vi "Camera ROI.vi"(10 "View (%)":sgl=100.0 min=0 max=100, 11 "Crop Point":i32=60 min=0 max=160 step=1) -> (3 "Camera ROI":i32[](array[numeric]))   [LabVIEW 2012]
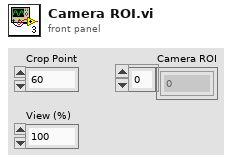
[diagram p1: front panel]
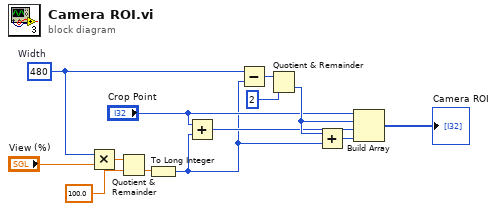
[diagram p0: block diagram]
diagram:
  w5 = 480  # Width
  n1 = Multiply(x=w5, y="View (%)") -> (x*y=w4:sgl)
  n2 = Quotient & Remainder(x=w4, y=sgl 100.0) -> (floor(x/y)=w2:sgl)  [unwired: 1 out]
  n3 = To Long Integer(number=w2) -> (32bit integer=w1:i32)
  n4 = Add(x="Crop Point", y=w1) -> (x+y=w8:i32)
  n5 = Subtract(x=w5, y=w1) -> (x-y=w10:i32)
  n6 = Quotient & Remainder(x=w10, y=2) -> (floor(x/y)=w13:i32)  [unwired: 1 out]
  n7 = Add(x=w13, y=w1) -> (x+y=w12:i32)
  n8 = Build Array("Crop Point", w13, w8, w12) -> (→"Camera ROI":i32[])
